vi "Construct Listbox Bus Monitor Panel.vi"(10 "Show Panel Boolean":string) -> (3 "ListboxBusMonitorPanel out":refnum<class "ListboxBusMonitorPanel.lvclass">)   [LabVIEW 2020, in "MVA Framework.lvlib" / "ListboxBusMonitor.lvlib" / "ListboxBusMonitorPanel.lvclass"]
doc: "构建列表框总线监控面板"
uses:
  ListboxBusMonitorPanel.lvclass
  ListboxBusMonitorPanel.lvclass/ListboxBusMonitorPanel.ctl
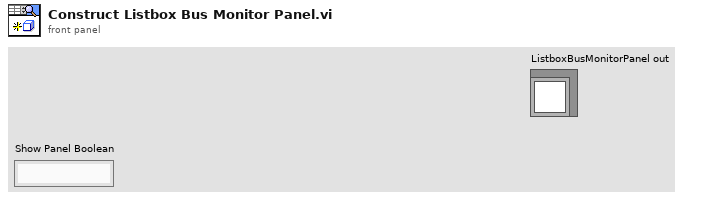
[diagram p1: front panel]
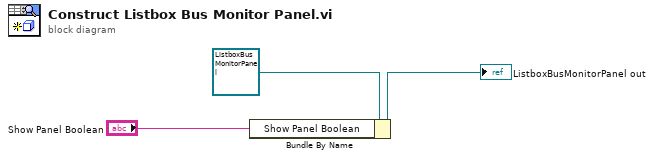
[diagram p0: block diagram]
diagram:
  n1 = Bundle By Name(cluster=refnum<class "ListboxBusMonitorPanel.lvclass"> refnum ("ListboxBusMonitorPanel in"), "Show Panel Boolean"="Show Panel Boolean") -> (→"ListboxBusMonitorPanel out":refnum<class "ListboxBusMonitorPanel.lvclass">)
